vi "Global Value 1.vi"   [LabVIEW 2015]
uses:
  <vilib>/rvi/Emulation/niFpgaSctlEmulationGetInTimedLoop.vi
  Globals/Global_Sample per Frame.vi
  <vilib>/rvi/Emulation/niFpgaProcessEmulError.vi
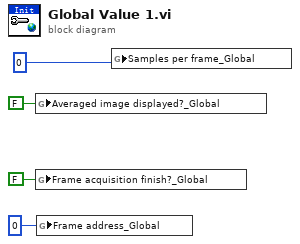
[diagram p0: block diagram]
diagram:
  n1 = global write "Global_Sample per Frame.vi" "Averaged image displayed?_Global"(FALSE ("Averaged image displayed?")) -> ()
  n2 = global write "Global_Sample per Frame.vi" "Frame acquisition finish?_Global"(FALSE ("Frame acquisition finish?")) -> ()
  n3 = global write "Global_Sample per Frame.vi" "Frame address_Global"(u32 0 ("Frame address")) -> ()
  n4 = global write "Global_Sample per Frame.vi" "Samples per frame_Global"(u32 0 ("Samples per frame_Global")) -> ()
